vi "Build State List.vi"(10 "Device Info":T2={"Devices"=[], "Pin Information"={"List of IO Names"=["sbRIO-9651 Socket\\PMOD1_Pin4_out", "sbRIO-9651 Socket\\PMOD1_Pin3_in", "sbRIO-9651 Socket\\PMOD1_Pin2_out", "sbRIO-9651 Socket\\PMOD1_Pin1_out"], "List of Enable Lines"=["sbRIO-9651 Socket\\PMOD1_Pin4_enable", "sbRIO-9651 Socket\\PMOD1_Pin3_enable", "sbRIO-9651 Socket\\PMOD1_Pin2_enable", "sbRIO-9651 Socket\\PMOD1_Pin1_enable"]}, "Replacement VI for DLU"=path "", "Replacement VI for SPI Engine"=path ""}) -> (2 "State List":T1[](array[typedef]))   [LabVIEW 2014, in "SPI Engine Scripting.lvlib"]
doc: "Builds a State List for each bus to be scripted. The lists are built using data from the Device Info input. The states in this list will be executed by the state machine in sequential order."
uses:
  SPI Engine Scripting.lvlib
  Controls/Bus Information.ctl
  Controls/Device Information.ctl
  <vilib>/LabVIEW Icon API/API_Text.ctl
  Controls/Pin Information.ctl
  Scripting States.ctl
  <vilib>/LabVIEW Icon API/LabVIEW Icon API.lvlib
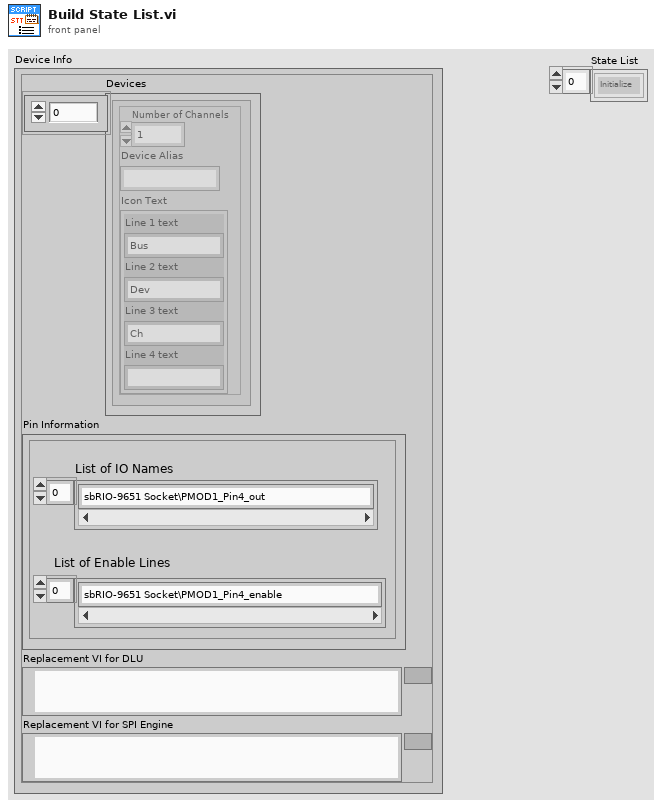
[diagram p1: front panel]
types:
  T1 = typedef "Scripting States.ctl" = enum16{"Initialize", "Copy Template Bus Directory", "Modify Dequeue Commands", "Modify Enqueue Data", "Create FPGA VI", "Create Project FIFOs", "Create FPGA Data Nodes", "Place FPGA Data Nodes", "Update Node Count in Engine", "Expand FIFO Type Def", "Populate FIFO Names in Engine", "Modify I/O Pin Names", "Modify I/O Pin Enable", "Replace DLU", "Add Engine to Project", "Place SPI Engine", "Scripting Complete Check", "End"}
  T2 = typedef "SPI Engine Scripting.lvlib/Bus Information.ctl" = cluster{"Devices":T3[], "Pin Information":T5, "Replacement VI for DLU":path, "Replacement VI for SPI Engine":path}
  T3 = typedef "Device Information.ctl" = cluster{"Number of Channels":i32, "Device Alias":string, "Icon Text":T4}
  T4 = typedef "LabVIEW Icon API.lvlib/API_Text.ctl" = cluster{"Line 1 text":string, "Line 2 text":string, "Line 3 text":string, "Line 4 text":string}
  T5 = typedef "Pin Information.ctl" = cluster{"List of IO Names":string[], "List of Enable Lines":string[]}
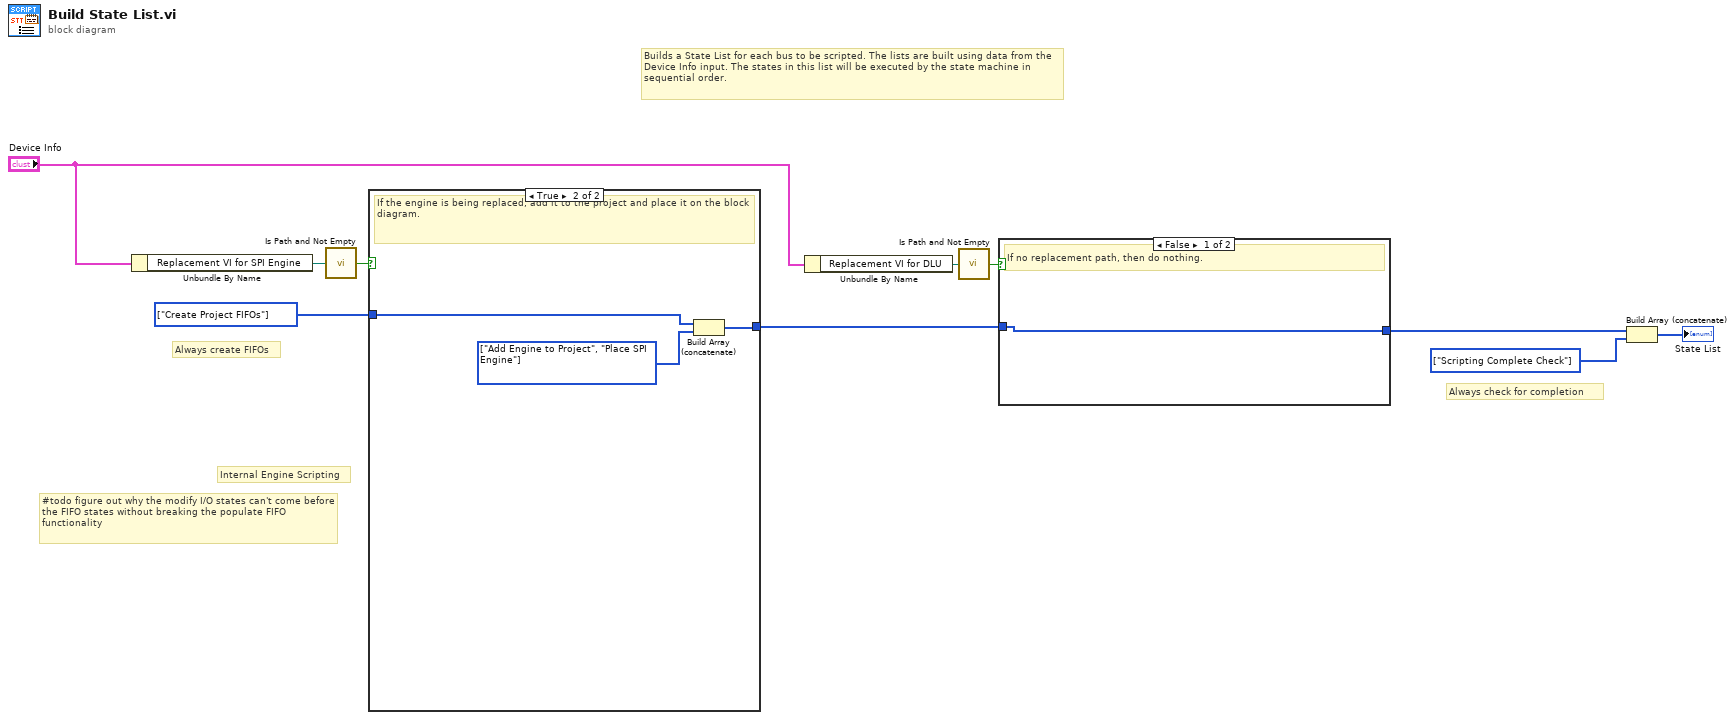
[diagram p0: block diagram]
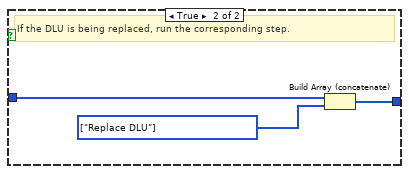
[diagram p2: hidden frame]
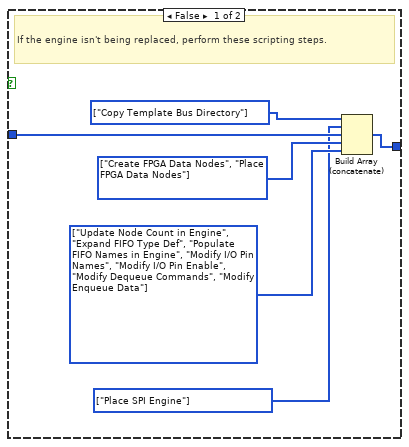
[diagram p3: hidden frame]
diagram:
  w2 = T1[] [enum."Scripting Complete Check"] items=["Initialize", "Copy Template Bus Directory", "Modify Dequeue Commands", "Modify Enqueue Data", "Create FPGA VI", "Create Project FIFOs", "Create FPGA Data Nodes", "Place FPGA Data Nodes", "Update Node Count in Engine", "Expand FIFO Type Def", "Populate FIFO Names in Engine", "Modify I/O Pin Names", "Modify I/O Pin Enable", "Replace DLU", "Add Engine to Project", "Place SPI Engine", "Scripting Complete Check", "End"]
  w9 = T1[] [enum."Create Project FIFOs"] items=["Initialize", "Copy Template Bus Directory", "Modify Dequeue Commands", "Modify Enqueue Data", "Create FPGA VI", "Create Project FIFOs", "Create FPGA Data Nodes", "Place FPGA Data Nodes", "Update Node Count in Engine", "Expand FIFO Type Def", "Populate FIFO Names in Engine", "Modify I/O Pin Names", "Modify I/O Pin Enable", "Replace DLU", "Add Engine to Project", "Place SPI Engine", "Scripting Complete Check", "End"]
  # "#todo figure out why the modify I/O states can't come before the FIFO states without breaking the populate FIFO functionality"
  # "Builds a State List for each bus to be scripted. The lists are built using data from the Device Info input. The states in this list will be executed by the state machine in sequential order."
  # "Always check for completion"
  # "Internal Engine Scripting"
  # "Always create FIFOs"
  n1 = Unbundle By Name("Device Info") -> ("Replacement VI for SPI Engine"=w10:path)
  n2 = call <vilib>:"Is Path and Not Empty.vi"("path"=w10) -> ("Is Path and Not Empty?"=w8:bool)  [unwired: 4 in]
  n3 = case shown="True" w8 {
    tunnel: w9 -> [w16 w19]
    tunnel: [w13 w18] -> w5
    frame False {
      w11 = T1[] [enum."Copy Template Bus Directory"] items=["Initialize", "Copy Template Bus Directory", "Modify Dequeue Commands", "Modify Enqueue Data", "Create FPGA VI", "Create Project FIFOs", "Create FPGA Data Nodes", "Place FPGA Data Nodes", "Update Node Count in Engine", "Expand FIFO Type Def", "Populate FIFO Names in Engine", "Modify I/O Pin Names", "Modify I/O Pin Enable", "Replace DLU", "Add Engine to Project", "Place SPI Engine", "Scripting Complete Check", "End"]
      w12 = T1[] [enum."Place SPI Engine"] items=["Initialize", "Copy Template Bus Directory", "Modify Dequeue Commands", "Modify Enqueue Data", "Create FPGA VI", "Create Project FIFOs", "Create FPGA Data Nodes", "Place FPGA Data Nodes", "Update Node Count in Engine", "Expand FIFO Type Def", "Populate FIFO Names in Engine", "Modify I/O Pin Names", "Modify I/O Pin Enable", "Replace DLU", "Add Engine to Project", "Place SPI Engine", "Scripting Complete Check", "End"]
      w14 = T1[] [enum."Update Node Count in Engine", enum."Expand FIFO Type Def", enum."Populate FIFO Names in Engine", enum."Modify I/O Pin Names", enum."Modify I/O Pin Enable", enum."Modify Dequeue Commands", enum."Modify Enqueue Data"] items=["Initialize", "Copy Template Bus Directory", "Modify Dequeue Commands", "Modify Enqueue Data", "Create FPGA VI", "Create Project FIFOs", "Create FPGA Data Nodes", "Place FPGA Data Nodes", "Update Node Count in Engine", "Expand FIFO Type Def", "Populate FIFO Names in Engine", "Modify I/O Pin Names", "Modify I/O Pin Enable", "Replace DLU", "Add Engine to Project", "Place SPI Engine", "Scripting Complete Check", "End"]
      w15 = T1[] [enum."Create FPGA Data Nodes", enum."Place FPGA Data Nodes"] items=["Initialize", "Copy Template Bus Directory", "Modify Dequeue Commands", "Modify Enqueue Data", "Create FPGA VI", "Create Project FIFOs", "Create FPGA Data Nodes", "Place FPGA Data Nodes", "Update Node Count in Engine", "Expand FIFO Type Def", "Populate FIFO Names in Engine", "Modify I/O Pin Names", "Modify I/O Pin Enable", "Replace DLU", "Add Engine to Project", "Place SPI Engine", "Scripting Complete Check", "End"]
      # "If the engine isn't being replaced, perform these scripting steps."
      n4 = Build Array (concatenate)(w11, w12, w16, w15, w14) -> (w13:T1[])
    }
    frame True {
      w17 = T1[] [enum."Add Engine to Project", enum."Place SPI Engine"] items=["Initialize", "Copy Template Bus Directory", "Modify Dequeue Commands", "Modify Enqueue Data", "Create FPGA VI", "Create Project FIFOs", "Create FPGA Data Nodes", "Place FPGA Data Nodes", "Update Node Count in Engine", "Expand FIFO Type Def", "Populate FIFO Names in Engine", "Modify I/O Pin Names", "Modify I/O Pin Enable", "Replace DLU", "Add Engine to Project", "Place SPI Engine", "Scripting Complete Check", "End"]
      # "If the engine is being replaced, add it to the project and place it on the block diagram."
      n5 = Build Array (concatenate)(w19, w17) -> (w18:T1[])
    }
  }
  n6 = Unbundle By Name("Device Info") -> ("Replacement VI for DLU"=w7:path)
  n7 = call <vilib>:"Is Path and Not Empty.vi"("path"=w7) -> ("Is Path and Not Empty?"=w4:bool)  [unwired: 4 in]
  n8 = case shown="False" w4 {
    tunnel: w5 -> [w20 w23]
    tunnel: [w20 w21] -> w3
    frame False {
      # "If no replacement path, then do nothing."
    }
    frame True {
      w22 = T1[] [enum."Replace DLU"] items=["Initialize", "Copy Template Bus Directory", "Modify Dequeue Commands", "Modify Enqueue Data", "Create FPGA VI", "Create Project FIFOs", "Create FPGA Data Nodes", "Place FPGA Data Nodes", "Update Node Count in Engine", "Expand FIFO Type Def", "Populate FIFO Names in Engine", "Modify I/O Pin Names", "Modify I/O Pin Enable", "Replace DLU", "Add Engine to Project", "Place SPI Engine", "Scripting Complete Check", "End"]
      # "If the DLU is being replaced, run the corresponding step."
      n9 = Build Array (concatenate)(w23, w22) -> (w21:T1[])
    }
  }
  n10 = Build Array (concatenate)(w3, w2) -> (→"State List":T1[])
